vi "Scale TDMS Data.vi"() -> ()   [LabVIEW 2023]
doc: "This example demonstrates how to create scaling information on TDMS objects (channel/group/root) using the TDMS Create Scaling Information VI and how to read the scaled data."
uses:
  <vilib>/Utility/tdmsutil.llb/TDMS Create Scaling Information (Linear).vi
  <vilib>/Utility/TDMS File Viewer/NI_TDMS File Viewer.lvlib
panel:
  in  "y intercept 2":dbl=5.0
  in  "slope 2":dbl=4.0
  in  "y intercept 1":dbl=3.0
  in  "slope 1":dbl=2.0
  out "Waveform Graph":waveform(dbl)[](graph)
  # "Overview: Demonstrates how to create scaling information on .tdms file objects (channel/group/root) using the TDMS Create Scaling Information VI and how to read the scaled data.\nInstructions:\n1. Run the VI.\n2. Delete the .tdms file (located at [LabVIEW Data]\\Example Scaling.tdms) when you are done."
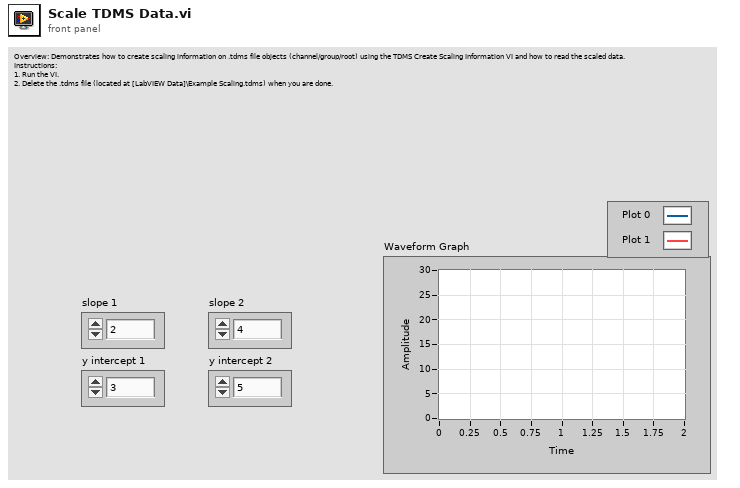
[diagram p1: front panel]
types:
  T1 = cluster{"slope":dbl, "y intercept":dbl, "input source":i32}
  T2 = enum16{"open", "open or create", "create or replace", "create", "open (read-only)"}
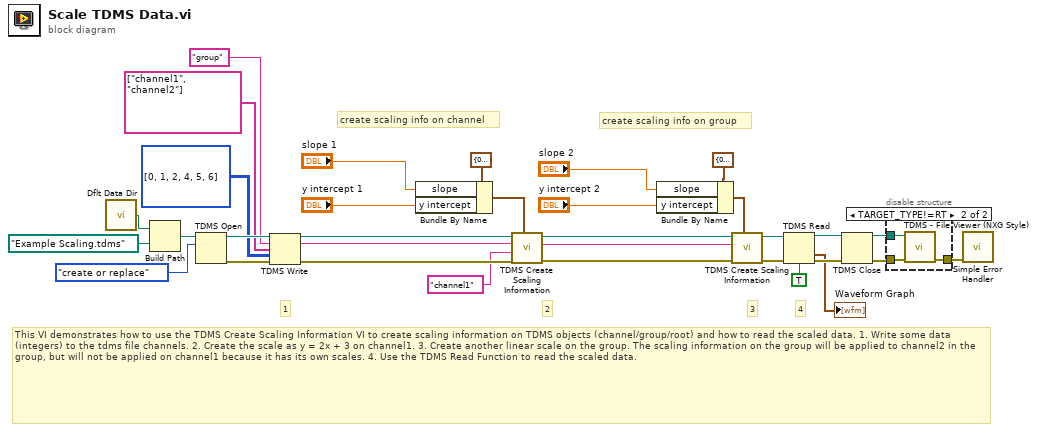
[diagram p0: block diagram]
diagram:
  # "4"
  # "3"
  # "2"
  # "1"
  # "create scaling info on channel"
  # "This VI demonstrates how to use the TDMS Create Scaling Information VI to create scaling information on TDMS objects (channel/group/root) and how to read the scaled data. 1. Write some data (integers) to the tdms file channels. 2. Create the scale as y = 2x + 3 on channel1. 3. Create another linear scale on the group. The scaling information on the group will be applied to channel2 in the group, but will not be applied on channel1 because it has its own scales. 4. Use the TDMS Read Function to read the scaled data."
  # "create scaling info on group"
  n1 = call <vilib>:"Dflt Data Dir.vi"() -> ("App:Default Data Directory"=w13:path)
  n2 = Build Path(base path=w13, name or relative path=path "Example Scaling.tdms" ("file path")) -> (appended path=w12:path)
  n3 = TDMS Open(10:T2."create or replace" ("operation"), 11:w12) -> (0:w31:errorcluster, 3:w32:refnum<k34>)  [unwired: 5 in]
  n4 = TDMS Write(0:w32, 5:"group" ("group name in (Untitled)"), 7:string[] ["channel1", "channel2"] ("channel name(s) in (Untitled)"), 9:i32[][] [[0, 1, 2], [4, 5, 6]], 11:w31) -> (4:w27:refnum<k34>, 6:w25:string, 15:w26:errorcluster)  [unwired: 1 in, 1 out]
  n5 = Bundle By Name(cluster=T1 {"slope"=0.0, "y intercept"=0.0, "input source"=-1} ("linear scale"), "slope"="slope 1", "y intercept"="y intercept 1") -> (w7:T1)
  n6 = call-poly <vilib>:"TDMS Create Scaling Information.vi"("linear scale"=w7, "error in (no error)"=w26, "channel name"="channel1", "group name"=w25, "tdms file"=w27) -> ("error out"=w21:errorcluster, "group name out"=w22:string, "tdms file out"=w23:refnum<k34>)  [unwired: 2 in, 2 out]
  n7 = Bundle By Name(cluster=T1 {"slope"=0.0, "y intercept"=0.0, "input source"=-1} ("linear scale"), "slope"="slope 2", "y intercept"="y intercept 2") -> (w3:T1)
  n8 = call-poly <vilib>:"TDMS Create Scaling Information.vi"("linear scale"=w3, "error in (no error)"=w21, "group name"=w22, "tdms file"=w23) -> ("error out"=w19:errorcluster, "tdms file out"=w20:refnum<k34>)  [unwired: 3 in, 3 out]
  n9 = TDMS Read(0:w20, 11:w19, 13:TRUE ("return channels in file order? (F)")) -> (4:w16:refnum<k34>, 10:→"Waveform Graph":waveform(dbl)[], 15:w17:errorcluster)  [unwired: 5 in, 3 out]
  n10 = TDMS Close(8:w17, 11:w16) -> (0:w10:errorcluster, 3:w11:path)
  n11 = disable-structure shown="TARGET_TYPE!=RT" {
    disable-tunnel: w10 -> [w34 w37]
    disable-tunnel: w11 -> [_ w36]
    disable-tunnel: [w34 w35] -> w9
    frame condition #0 {
    }
    frame condition #1 (active) {
      n12 = call <vilib>:"TDMS - File Viewer (NXG Style).vi"("error in"=w37, "file in"=w36) -> ("error out"=w35:errorcluster)  [unwired: 8 in, 1 out]
    }
  }
  n13 = call <vilib>:"Simple Error Handler.vi"("error in (no error)"=w9) -> ()  [unwired: 4 in, 5 out]
